vi "Visibility Timeout Helper.vi"(5 "Update?":bool, 7 "Visible":bool, 11 "Visible Timeout mS":i32) -> (3 "Timeout":i32)   [LabVIEW 2014, in "OOPanel.lvlib" / "Panel.lvclass"]
uses:
  Panel.lvclass
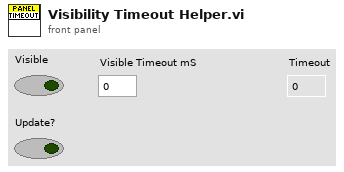
[diagram p1: front panel]
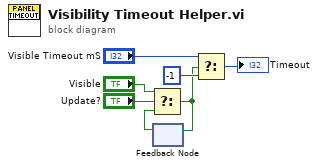
[diagram p0: block diagram]
diagram:
  n1 = feedback #1() -> (w2:bool)  [unwired: 1 in]
  n2 = Select(t="Visible", s="Update?", f=w2) -> (s? t:f=w1:bool)
  n3 = feedback-in #1(w1) -> ()
  n4 = Select(t="Visible Timeout mS", s=w1, f=-1) -> (s? t:f=→"Timeout":i32)
